vi "Read Initial.vi"(0 "VISA resource name":refnum<visa-resource-name>="COM1", 5 "write":bool=TRUE, 6 "read":bool=TRUE) -> (8 "string to write":string="*IDN?\n", 9 "read string":string, 10 "bytes read":u32)   [LabVIEW 2012]
doc: "The Basic Serial Read and Write example performs a Serial Port Read, a Serial Port Write, or a combination of these actions. The user selects the actions (read or write) on the front panel. If both are selected, the VI will write the data first, read data, and then close the VISA session that is opened to the port. This VI will wait until the specified number of bytes is received at the port or until a termination character is read.\n\nINSTRUCTIONS:\n1) Select the serial resource and configuration parameters (baud rate, data bits, parity, stop bits, flow control).\n2) Select the operations to be performed. \n3) Connect the serial port to your device. If no device is available, perform a loopback test by doing one of the following. Short pins 2 and 3 on a RS-232 cable or short pin 4 to pin 8 and pin 5 to pin 9 on a RS-485/422 cable. \n4) Run the VI to see the data read. (The \"read string\" will match the \"string to write\" if a loopback test was performed.)\n\nNote: The parameters set for the serial port must match the parameters of the connected instrument or device. In this example, the bytes to read parameter specifies the number of bytes that the serial port reads. If there were more bytes at the port than the number specified in bytes to read, those bytes would not be read. Also, if you specify to read more bytes than the number of bytes actually read, you might receive a timeout error message.\n\nOn the block diagram, the Configure Serial Port VI sets the configuration parameters. The front panel displays the controls used to configure the basic parameters, such as baud rate, data bits, and parity. Constants configure the other parameters the user probably does not need set. After the VISA Configure Serial Port VI opens the VISA session and configures the port, the VI passes the VISA resource name to other VIs that perform operations on that VISA resource. The VISA Write function sends a command to the serial device and the VISA Read function returns data based on the command. The VISA Close function then closes the reference to the serial device. It is important to close the reference; otherwise communication through with that port through protocols other than VISA might not be possible."
uses:
  <vilib>/Instr/_visa.llb/VISA Configure Serial Port (Instr).vi
panel:
  out "Numeric":i32
  in  "length (rest)":i32
  in  "Offset":string
  in  "Data":string
  in  "Length":u8
  in  "Offset":i8[](array[numeric]) format="%x"
  in  "Page":i8 min=0 max=3 step=1
  in  "Write":bool
  in  "Addr":i8 min=0 max=15 step=1
  in  "delay before read (ms)":u32=500
  # "Select the serial resource and the operations (Read, Write, or both) to be performed.  If both are selected, the VI will write the data first, read data and then close the VISA session that is opened to the port.  This VI will wait until the specified number of bytes is received at the port or until a termination character is read."
  # "For additional information select File >> VI Properties >> Documentation"
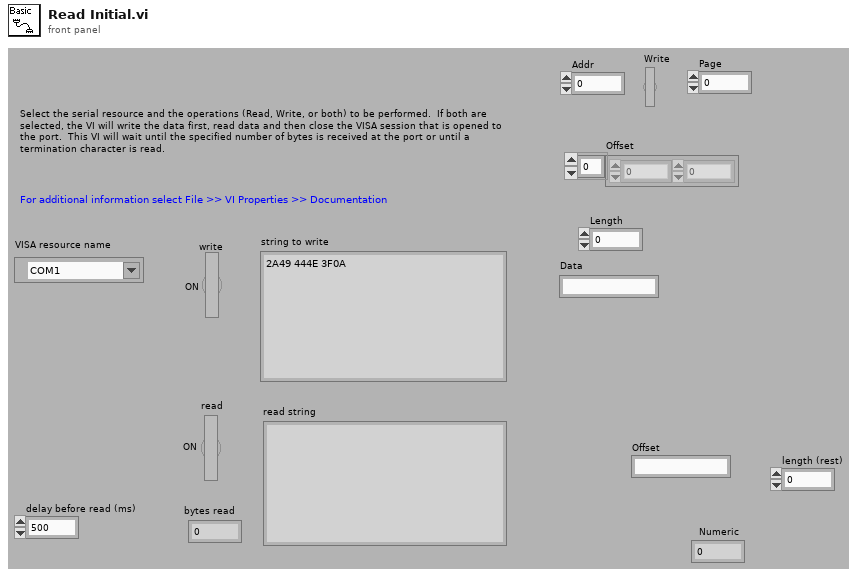
[diagram p1: front panel]
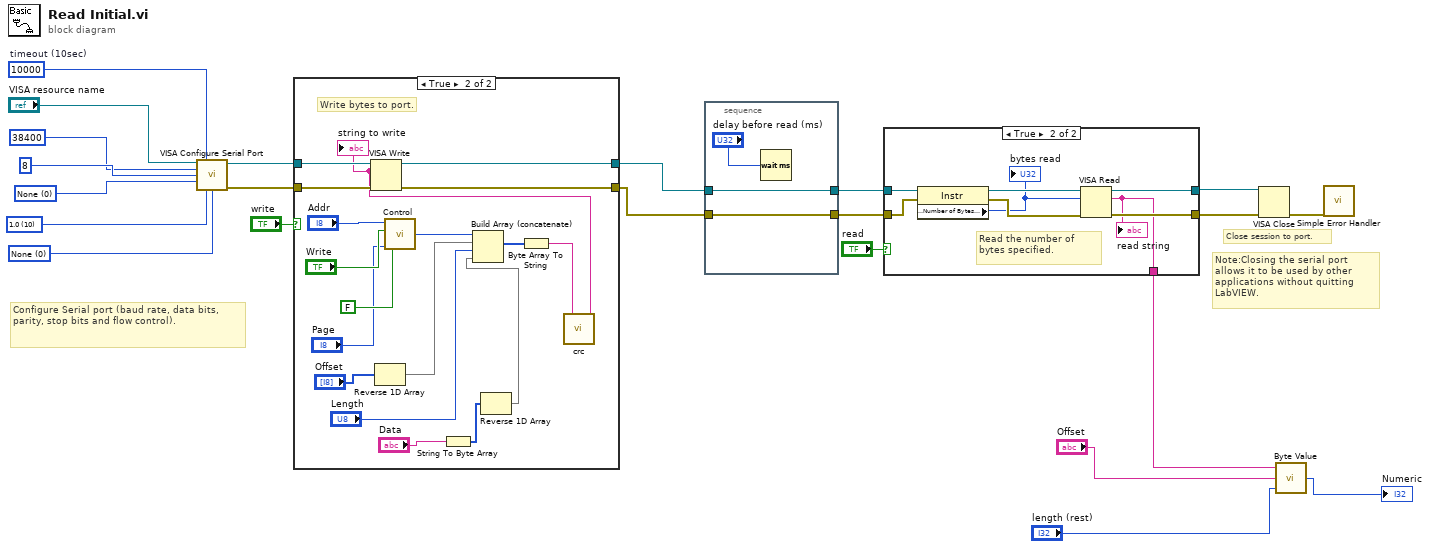
[diagram p0: block diagram]
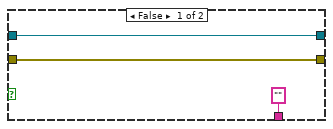
[diagram p3: hidden frame]
diagram:
  w12 = u16 0 items=["None"=0, "XON/XOFF"=1, "RTS/CTS"=2, "DTR/DSR"=4] ("flow control")
  w13 = u16 10 items=["1.0"=10, "1.5"=15, "2.0"=20] ("stop bits")
  w15 = u16 0 items=["None", "Odd", "Even", "Mark", "Space"] ("parity")
  w14 = u32 10000  # timeout (10sec)
  # "Note:Closing the serial port allows it to be used by other applications without quitting LabVIEW."
  # "Configure Serial port (baud rate, data bits, parity, stop bits and flow control)."
  # "Close session to port."
  n1 = call-poly "VISA Configure Serial Port"("VISA resource name"="VISA resource name", "timeout (10sec)"=w14, "baud rate (9600)"=u32 38400, "data bits (8)"=u16 8 ("data bits"), "parity (0:none)"=w15, "stop bits (10: 1 bit)"=w13, "flow control (0:none)"=w12) -> ("VISA resource name out"=w19:refnum<visa-resource-name>, "error out"=w20:errorcluster)  [unwired: 2 in, 5 out]
  n2 = case shown="True" "write" {
    tunnel: [w24 w42] -> w9
    tunnel: w19 -> [w23 w41]
    tunnel: w20 -> [w24 w40]
    tunnel: [w23 w39] -> w7
    frame False {
    }
    frame True {
      # "Write bytes to port."
      n3 = Reverse 1D Array(array="Offset") -> (reversed array=w32:i8[])
      n4 = call "Control.vi"("Page"="Page", "Error"=FALSE, "Write"="Write", "Addr"="Addr") -> ("Control Byte"=w34:u32)
      n5 = String To Byte Array(string="Data") -> (unsigned byte array=w29:u8[])
      n6 = Reverse 1D Array(array=w29) -> (reversed array=w28:u8[])
      n7 = Build Array (concatenate)(w34, w32, "Length", w28) -> (w27:u32[])
      n8 = Byte Array To String(unsigned byte array=w27) -> (string=w26:string)
      n9 = call "crc.vi"("Input string"=w26) -> ("Output (with crc)"=w25:string)
      "string to write" <- w25
      n10 = VISA Write(VISA resource name=w41, write buffer=w25, error in (no error)=w40) -> (VISA resource name out=w39:refnum<visa-resource-name>, error out=w42:errorcluster)  [unwired: 1 out]
    }
  }
  n11 = stacked-sequence {
    tunnel: w9 -> [w45]
    tunnel: [w45] -> w8
    tunnel: w7 -> [w44]
    tunnel: [w44] -> w6
    frame #0 {
      n12 = Wait (ms)(milliseconds to wait="delay before read (ms)") -> ()  [unwired: 1 out]
    }
  }
  n13 = case shown="True" "read" {
    tunnel: w8 -> [w48 w52]
    tunnel: [w48 w56] -> w18
    tunnel: [w47 w55] -> w17
    tunnel: w6 -> [w47 w54]
    tunnel: ["" ("read buffer") w49] -> w4
    frame False {
    }
    frame True {
      # "Read the number of bytes specified."
      n14 = property class="Instr"(reference=w54, error in=w52) -> (reference out=w53:refnum<visa-resource-name>, error out=w51:errorcluster, "Serial Settings:Number of Bytes at Serial Port"=w50:u32)
      "bytes read" <- w50
      n15 = VISA Read(VISA resource name=w53, byte count=w50, error in (no error)=w51) -> (VISA resource name out=w55:refnum<visa-resource-name>, read buffer=w49:string, error out=w56:errorcluster)  [unwired: 1 out]
      "read string" <- w49
    }
  }
  n16 = VISA Close(VISA resource name=w17, error in (no error)=w18) -> (error out=w16:errorcluster)
  n17 = call "Byte Value.vi"("Length"="length (rest)", "Offset"="Offset", "string"=w4) -> ("Value"=→"Numeric":i32)
  n18 = call <vilib>:"Simple Error Handler.vi"("error in (no error)"=w16) -> ()  [unwired: 1 in, 8 out]
